vi "Untitled 5.vi"() -> ()   [LabVIEW 2012]
panel:
  out "error out":errorcluster
  in  "Expression":string
  out "Result":dbl
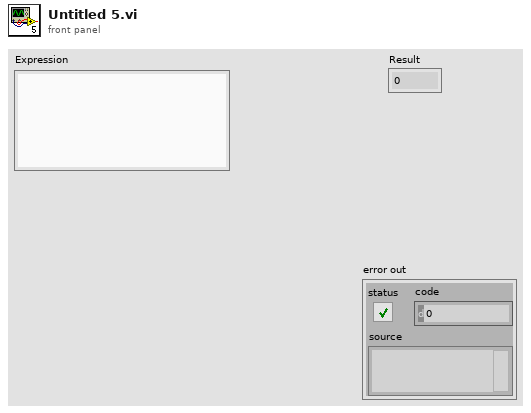
[diagram p1: front panel]
types:
  T1 = cluster{"String":string, "avgs":cluster{"Expression":string, "Durration":dbl, "Replacement":string, "Values":dbl[]}[]}
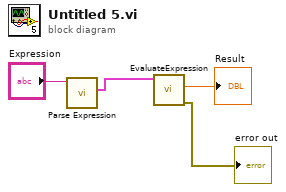
[diagram p0: block diagram]
diagram:
  n1 = call "Parse Expression.vi"("Expression"="Expression") -> ("Parsed Expression"=w4:T1)  [unwired: 9 in, 1 out]
  n2 = call "EvaluateExpression.vi"("Parsed Expression"=w4) -> ("error out"=→"error out":errorcluster, "Result"=→"Result":dbl)  [unwired: 9 in]
